vi "WriteSizeMat_1DArray_U8.vi"(6 "Channel":i32=1, 8 "error in":errorcluster, 9 "Height":i32, 10 "Width":i32, 11 "Array in":u8[](array[numeric])) -> (0 "error out":errorcluster, 3 "Array out":u8[](array[numeric]))   [LabVIEW 2020, in "OpenLvVision_OpenCv.lvlib"]
doc: "Write size of the datatype\nNo malleable to breake vi inlining!"
uses:
  OpenLvVision_OpenCv.lvlib
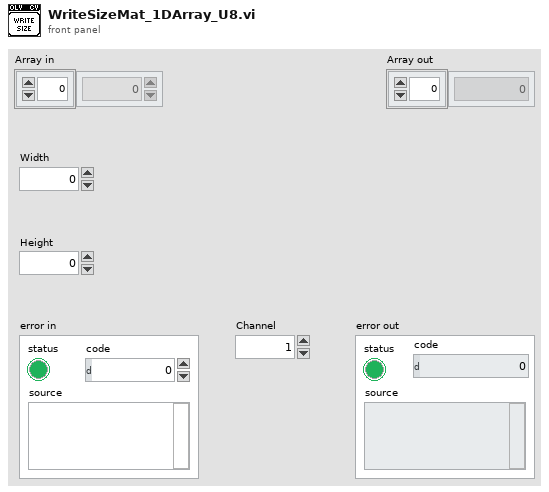
[diagram p1: front panel]
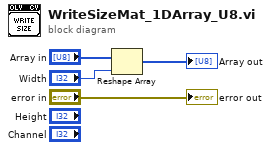
[diagram p0: block diagram]
diagram:
  n1 = Reshape Array("Array in", "Width") -> (→"Array out":u8[])
  "error out" <- "error in"
